vi "HFRR ADV v12.vi"() -> ()   [LabVIEW 2025] (continued)
            n428 = call "IMAGE PATH CREATION PY.vi"("error in (no error)"=w659, "File Name :"=w660) -> ("error out"=w658:errorcluster, "File Path"=w646:path, "File Path String:"=w641:string)  [unwired: 7 in]
            n429 = Match Pattern(string=w654, regular expression=",") -> (before substring=w640:string)  [unwired: 1 in, 3 out]
            n430 = local read "Calibration Tab"() -> (w643:enum32{"Measrument", "Calibrate"})
            n431 = call "Stall Data Flow.vim"("value in"=w658, "milliseconds to wait"=u32 250) -> ("value out"=w642:errorcluster)  [unwired: 1 out]
            n432 = Equal?(x=w640, y="\"rectangle\"") -> (x = y?=w651:bool)
            n433 = case shown="False" w651 {
              tunnel: w650 -> [w705 w760]
              tunnel: w647 -> [_ w751]
              tunnel: cluster{"major":dbl, "minor":dbl, "average":dbl} {"major"=0.0, "minor"=0.0, "average"=0.0} -> [w703 w747]
              tunnel: [w702 w744] -> w645
              tunnel: w640 -> [w704 _]
              tunnel: w647 -> [w701 _]
              frame False {
                n434 = Equal?(x=w704, y="\"line\"") -> (x = y?=w706:bool)
                n435 = case shown="True" w706 {
                  tunnel: w705 -> [_ w721]
                  tunnel: w703 -> [w708 w720]
                  tunnel: [w708 w718] -> w702
                  tunnel: w701 -> [_ w717]
                  frame False {
                  }
                  frame True {
                    w716 = 0.0 ("Major Axis")
                    n436 = Match Pattern(string=w721, regular expression="\"length_px\":") -> (after substring=w719:string)  [unwired: 1 in, 3 out]
                    n437 = property on="Major Axis" class="DigNum (strict)"("Caption.Text"="") -> ()  [unwired: 2 in, 2 out]
                    n438 = property on="Minor Axis" class="DigNum (strict)"("Caption.Text"="") -> ()  [unwired: 2 in, 2 out]
                    n439 = property on="Average" class="DigNum (strict)"("Caption.Text"="Line") -> ()  [unwired: 2 in, 2 out]
                    n440 = Fract/Exp String To Number(string=w719, default (0 dbl)=0.0 ("default (0 DBL)")) -> (number=w715:dbl)  [unwired: 2 in, 1 out]
                    "Pixel Value" <- w715
                    n441 = Multiply(x=w715, y=w717) -> (x*y=w728:dbl)
                    n442 = Multiply(x=w728, y=1000.0) -> (x*y=w711:dbl)
                    n443 = Divide(x=w711, y=1000.0) -> (x/y=w714:dbl)
                    n444 = local write "Measurment (mm)"(w714) -> ()
                    n445 = Bundle By Name(cluster=w720, "average"=w711) -> (w718:cluster{"major":dbl, "minor":dbl, "average":dbl})
                    n446 = Number To Fractional String(number=w711, precision (6)=i16 1) -> (F-format string=w710:string)  [unwired: 2 in]
                    n447 = local write "Minor Axis"(w716) -> ()
                    n448 = local write "Major Axis"(w716) -> ()
                    n449 = Fract/Exp String To Number(string=w710) -> (number=w709:dbl)  [unwired: 3 in, 1 out]
                    n450 = local write "Average"(w709) -> ()
                  }
                }
              }
              frame True {
                w748 = 1000.0 ("y")
                w754 = 0.0 ("default (0 DBL)")
                n451 = Match Pattern(string=w760, regular expression=" \"width_px\":") -> (after substring=w758:string)  [unwired: 1 in, 3 out]
                n452 = Match Pattern(string=w758, regular expression="\"height_px\":") -> (before substring=w756:string, after substring=w755:string)  [unwired: 1 in, 2 out]
                n453 = Fract/Exp String To Number(string=w756, default (0 dbl)=w754) -> (number=w753:dbl)  [unwired: 2 in, 1 out]
                n454 = Fract/Exp String To Number(string=w755, default (0 dbl)=w754) -> (number=w752:dbl)  [unwired: 2 in, 1 out]
                n455 = Multiply(x=w753, y=w751) -> (x*y=w750:dbl)
                n456 = Multiply(x=w752, y=w751) -> (x*y=w749:dbl)
                n457 = Multiply(x=w750, y=w748) -> (x*y=w734:dbl)
                n458 = Multiply(x=w749, y=w748) -> (x*y=w732:dbl)
                n459 = Add(x=w734, y=w732) -> (x+y=w746:dbl)
                n460 = property on="Major Axis" class="DigNum (strict)"("Caption.Text"="Major Axis") -> ()  [unwired: 2 in, 2 out]
                n461 = property on="Minor Axis" class="DigNum (strict)"("Caption.Text"="Minor Axis") -> ()  [unwired: 2 in, 2 out]
                n462 = property on="Average" class="DigNum (strict)"("Caption.Text"="Average") -> ()  [unwired: 2 in, 2 out]
                n463 = Divide(x=w746, y=2.0) -> (x/y=w730:dbl)
                n464 = Bundle By Name(cluster=w747, "major"=w734, "minor"=w732, "average"=w730) -> (w744:cluster{"major":dbl, "minor":dbl, "average":dbl})
                n465 = Number To Fractional String(number=w732, precision (6)=i16 1) -> (F-format string=w739:string)  [unwired: 2 in]
                n466 = Number To Fractional String(number=w730, precision (6)=i16 1) -> (F-format string=w740:string)  [unwired: 2 in]
                n467 = Number To Fractional String(number=w734, precision (6)=i16 1) -> (F-format string=w738:string)  [unwired: 2 in]
                n468 = Fract/Exp String To Number(string=w739) -> (number=w731:dbl)  [unwired: 3 in, 1 out]
                n469 = Fract/Exp String To Number(string=w740) -> (number=w729:dbl)  [unwired: 3 in, 1 out]
                n470 = Fract/Exp String To Number(string=w738) -> (number=w733:dbl)  [unwired: 3 in, 1 out]
                n471 = local write "Major Axis"(w733) -> ()
                n472 = local write "Average"(w729) -> ()
                n473 = local write "Minor Axis"(w731) -> ()
              }
            }
            n474 = case shown="\"Measrument\", Default" w643 {
              tunnel: w646 -> [w673 _]
              tunnel: w645 -> [w672 _]
              tunnel: [w669 w698] -> w644
              tunnel: w642 -> [w671 w698]
              tunnel: w641 -> [w670 _]
              tunnel: w638 -> [w668 _]
              frame "Measrument", Default {
                n475 = stacked-sequence {
                  tunnel: w673 -> [w691 _]
                  tunnel: w672 -> [w689 _]
                  tunnel: w671 -> [w687 _]
                  tunnel: w670 -> [w686 _]
                  tunnel: [w681 _] -> w669
                  tunnel: w668 -> [w674 _]
                  frame #0 {
                    n476 = call "IMAGE ANALYSIS.vi"("Enum"=POST_ANALYSIS_ENUM."SAVE IMAGE", "error in"=w687, "IMAGE FILE PATH"=w686) -> ("error out"=w685:errorcluster)  [unwired: 7 in, 1 out]
                    n477 = call "Stall Data Flow.vim"("value in"=w685, "milliseconds to wait"=u32 1000) -> ("value out"=w676:errorcluster)  [unwired: 1 out]
                    n478 = local read "Test File List :"() -> (w693:string)
                    n479 = call "IMAGE ANALYSIS.vi"("Enum"=POST_ANALYSIS_ENUM."MINIMIZE UI", "error in"=w676) -> ("error out"=w683:errorcluster)  [unwired: 8 in, 1 out]
                    n480 = Bundle By Name(cluster=T21 {"File Name"="", "Test Method"="", "Operator"="", "Fuel Description"="", "Date and time"=""} ("Main Ref"), "Test Method"=w674, "File Name"=w693) -> (w694:T21)
                    n481 = call "Stall Data Flow.vim"("value in"=w683, "milliseconds to wait"=u32 1500) -> ("value out"=w678:errorcluster)  [unwired: 1 out]
                    n482 = call "duf file read.vi"("error in (no error)"=w678, "Main Ref"=w694) -> ("error out"=w692:errorcluster, "Main Ref 2"=w690:T21)  [unwired: 8 in]
                    n483 = call "DETECTION REPORT for manual.vi"("error in (no error)"=w692, "return value 3"=w689, "Image File Path"=w691, "Main Ref"=w690) -> ("error out"=w688:errorcluster)  [unwired: 7 in]
                    n484 = call <vilib>:"Clear Errors.vi"("error in (no error)"=w688) -> ("error out"=w679:errorcluster)  [unwired: 5 in, 1 out]
                    n485 = call "IMAGE ANALYSIS.vi"("Enum"=POST_ANALYSIS_ENUM."MINIMIZE UI", "error in"=w679) -> ("error out"=w681:errorcluster)  [unwired: 8 in, 1 out]
                  }
                  frame #1 {
                    n486 = local write "Main Tab"(T2."HOME" ("Main Tab")) -> ()
                    n487 = local write "Main Dashboard Buttons"(T1."Home" ("Main Dashboard Buttons")) -> ()
                  }
                }
              }
              frame "Calibrate" {
              }
            }
          }
          frame #2 {
            n488 = Not(x=w763) -> (.not. x?=w762:bool)
            n489 = local write "Confirm Measrurement"(w762) -> ()
            n490 = local read "Calibration Tab"() -> (w761:enum32{"Measrument", "Calibrate"})
            n491 = case shown="\"Measrument\", Default" w761 {
              frame "Measrument", Default {
                n492 = local write "Main Tab"(T2."HOME" ("Main Tab")) -> ()
              }
              frame "Calibrate" {
              }
            }
          }
        }
      }
    }
    n493 = local read "Humidity"() -> (w506:bool)
    n494 = local read "Save Change"() -> (w511:bool)
    n495 = local read "Calibrate"() -> (w512:bool)
    n496 = local read "Auto Start Test"() -> (w507:bool)
    n497 = case shown="True" w512 {
      selector: w512 -> [_ w619]
      frame False {
      }
      frame True {
        n498 = Not(x=w619) -> (.not. x?=w618:bool)
        n499 = local write "Calibrate"(w618) -> ()
        n500 = local write "Calibration Tab"(enum32{"Measrument", "Calibrate"}."Calibrate" ("Calibration Tab")) -> ()
      }
    }
    n501 = case shown="True" w511 {
      selector: w511 -> [_ w563]
      frame False {
      }
      frame True {
        n502 = stacked-sequence {
          tunnel: w563 -> [_ _ _ _ w617]
          frame #0 {
            n503 = call "IMAGE ANALYSIS.vi"("Enum"=POST_ANALYSIS_ENUM."HIDE UI") -> ()  [unwired: 9 in, 2 out]
          }
          frame #1 {
            n504 = local read "100x gain"() -> (w565:dbl)
            n505 = local read "10x Gain"() -> (w566:dbl)
            n506 = local read "5x Gain"() -> (w567:dbl)
            n507 = Number To Fractional String(number=w566, width (-)=i16 4, precision (6)=i16 7) -> (F-format string=w588:string)  [unwired: 1 in]
            n508 = Number To Fractional String(number=0.0, width (-)=i16 4, precision (6)=i16 7) -> (F-format string=w583:string)  [unwired: 1 in]
            n509 = Number To Fractional String(number=w565, width (-)=i16 4, precision (6)=i16 7) -> (F-format string=w571:string)  [unwired: 1 in]
            n510 = Number To Fractional String(number=w567, width (-)=i16 10 ("precision (6)"), precision (6)=i16 7) -> (F-format string=w597:string)  [unwired: 1 in]
            n511 = Concatenate Strings("[CH1]" ("string"), w597, " - 5x Gain" ("string"), "\r") -> (w587:string)
            n512 = Concatenate Strings("[CH2]" ("string"), w588, " - 10x Gain" ("string"), "\r") -> (w586:string)
            n513 = Concatenate Strings("[CH3]" ("string"), w583, " - 20x Gain" ("string"), "\r") -> (w577:string)
            n514 = Concatenate Strings("[CH4]" ("string"), w571, " - 100x Gain" ("string"), "\r") -> (w570:string)
            n515 = String To Path(string="C:\\LAB-IQ\\Image Calibrate v01.dcf") -> (path=w600:path)
            n516 = Concatenate Strings(w587, w586, w577, w570) -> (w585:string)
            n517 = call <vilib>:"Write Characters To File.vi"("append to file? (new file:F)"=FALSE, "character string"=w585, "file path (dialog if empty)"=w600) -> ()  [unwired: 2 in, 1 out]
          }
          frame #2 {
            n518 = String To Path(string="C:\\LAB-IQ\\Image Calibrate v01.dcf") -> (path=w603:path)
            n519 = Open/Create/Replace File ("Open File")(file path (use dialog)=w603) -> (refnum out=w604:refnum<file>)  [unwired: 5 in, 2 out]
            n520 = for {
              N: 4 -> [_]
              tunnel: w604 -> [w610]
              i -> [w606]
              n521 = Read from Text File ("Read File")(file (use dialog)=w610) -> (text=w611:string)  [unwired: 3 in, 3 out]
              n522 = String Subset(string=w611, offset (0)=6, length (rest)=10 ("length (rest)")) -> (substring=w607:string)
              n523 = Fract/Exp String To Number(string=w607) -> (number=w605:dbl)  [unwired: 3 in, 1 out]
              n524 = case shown="3" w606 {
                tunnel: w605 -> [w612 w613 _ w614 _]
                frame 0 {
                  n525 = local write "5x Gain"(w612) -> ()
                }
                frame 1 {
                  n526 = local write "10x Gain"(w613) -> ()
                }
                frame 2 {
                }
                frame 3 {
                  n527 = local write "100x gain"(w614) -> ()
                }
                frame 4, Default {
                }
              }
            }
          }
          frame #3 {
            n528 = call "IMAGE ANALYSIS.vi"("Enum"=POST_ANALYSIS_ENUM."SHOW UI") -> ()  [unwired: 9 in, 2 out]
          }
          frame #4 {
            n529 = Not(x=w617) -> (.not. x?=w616:bool)
            n530 = local write "Save Change"(w616) -> ()
          }
        }
      }
    }
    n531 = case shown="False" w507 {
      tunnel: w506 -> [w533 _]
      frame False {
        n532 = case shown="True" w533 {
          frame False {
          }
          frame True {
            n533 = local read "Set Humidity:"() -> (w537:dbl)
            n534 = local read "Set Humidity:"() -> (w540:dbl)
            n535 = local read "Humidity ( %RH )"() -> (w541:dbl)
            n536 = Subtract(x=w537, y=2.0) -> (x-y=w535:dbl)
            n537 = Add(x=w540, y=2.0) -> (x+y=w536:dbl)
            n538 = In Range and Coerce(upper limit=w536, x=w541, lower limit=w535) -> (In Range?=w534:bool)  [unwired: 1 out]
            n539 = case shown="True" w534 {
              frame False {
              }
              frame True {
                n540 = case shown="False" "Manual Humididty Reached" {
                  selector: "Manual Humididty Reached" -> [_ w544]
                  frame False {
                  }
                  frame True {
                    n541 = Not(x=w544) -> (.not. x?=w543:bool)
                    n542 = local write "Manual Humididty Reached"(w543) -> ()
                    n543 = local read "EVENT LOG"() -> (w546:string)
                    n544 = call "Event Log.vi"("Content"="Target Humidity reached", "EVENT LOG"=w546) -> ("EVENT LOG"=w545:string)  [unwired: 8 in, 1 out]
                    n545 = local write "EVENT LOG"(w545) -> ()
                  }
                }
              }
            }
          }
        }
      }
      frame True {
        n546 = local write "Manual Humididty Reached"(TRUE ("Manual Humididty Reached")) -> ()
      }
    }
    n547 = local read "Cap Live Image"() -> (w527:bool)
    n548 = local read "SCAR MEASURMENT"() -> (w530:enum32{"Auto Scar", "Manual Scar"})
    n549 = Wait (ms)(milliseconds to wait=u32 250) -> ()  [unwired: 1 out]
    n550 = Equal?(x=w530, y=enum32{"Auto Scar", "Manual Scar"}."Manual Scar" ("SCAR MEASURMENT")) -> (x = y?=w528:bool)
    n551 = And(x=w528, y=w527) -> (x .and. y?=w526:bool)
    n552 = case shown="True" w526 {
      selector: w526 -> [_ w842]
      frame False {
      }
      frame True {
        n553 = stacked-sequence {
          tunnel: [_ _ _ w857 _] -> _
          tunnel: w842 -> [_ _ _ _ w863]
          frame #0 {
            w843 = 0.0
            n554 = local write "Major Axis"(w843) -> ()
            n555 = local write "Minor Axis"(w843) -> ()
            n556 = local write "Average"(w843) -> ()
          }
          frame #1 {
            n557 = call "CAMERA LIVE FEED FGV.vi"("Enum - Menu"=CAMERA_LIVE_FEED_ENUM."CAMERA MINIMIZE") -> ()  [unwired: 9 in, 2 out]
          }
          frame #2 {
            n558 = local read "FILE 3"() -> (w851:string)
            n559 = call <vilib>:"Trim Whitespace.vi"("string"="C:\\LAB-IQ\\images\\") -> ("trimmed string"=w853:string)  [unwired: 1 in]
            n560 = String To Path(string=w853) -> (path=w852:path)
            n561 = Concatenate Strings(w851, ".png" ("string")) -> (w850:string)
            n562 = Build Path(base path=w852, name or relative path=w850) -> (appended path=w848:path)
            n563 = Path To String(path=w848) -> (string=w847:string)
            n564 = call "CAMERA LIVE FEED FGV.vi"("Enum - Menu"=CAMERA_LIVE_FEED_ENUM."CAMERA SAVE", "Image Path"=w847) -> ("error out"=w845:errorcluster)  [unwired: 8 in, 1 out]
            n565 = case shown="No Error" w845 {
              frame No Error {
                n566 = One Button Dialog(message="Image saved successfully") -> ()  [unwired: 1 in, 1 out]
              }
              frame Error {
              }
            }
          }
          frame #3 {
            n567 = call "LIST FILE NAMES.vi"() -> ("error out"=w859:errorcluster, "filenames"=w856:string[])  [unwired: 10 in]
            n568 = call "IMAGE ANALYSIS.vi"("Enum"=POST_ANALYSIS_ENUM."SHOW UI", "error in"=w859) -> ("error out"=w857:errorcluster)  [unwired: 8 in, 1 out]
            n569 = property on="Test File List :" class="CmbBox"("Strings[]"=w856) -> ()  [unwired: 2 in, 2 out]
          }
          frame #4 {
            (unwired) T22."Report" ("Main Dashboard Buttons")
            n570 = Not(x=w863) -> (.not. x?=w862:bool)
            n571 = local write "Zoom Factore"(0.0 ("Zoom Factore")) -> ()
            n572 = local write "Cap Live Image"(w862) -> ()
            n573 = local write "Main Tab"(T2."Adv Scar Report" ("Main Tab")) -> ()
            n574 = property on="Cap Live Image" class="Bool (strict)"("BoolText.Text"="Capture Image" ("Boolean Text.Text")) -> ()  [unwired: 2 in, 2 out]
            n575 = local write "Main Dashboard Buttons"(T1."Report" ("Main Dashboard Buttons")) -> ()
          }
        }
      }
    }
    n576 = local read "change Gain"() -> (w510:bool)
    n577 = local read "Back Square"() -> (w509:bool)
    n578 = case shown="True" w510 {
      selector: w510 -> [_ w554]
      frame False {
      }
      frame True {
        n579 = stacked-sequence {
          tunnel: w554 -> [_ w562]
          frame #0 {
            n580 = local read "Actual (µm)"() -> (w558:dbl)
            n581 = local read "Pixel Value"() -> (w557:dbl)
            n582 = local read "Magnification :"() -> (w556:string)
            n583 = Divide(x=w558, y=w557) -> (x/y=w555:dbl)
            n584 = case shown="\"10x\"" w556 {
              tunnel: w555 -> [w559 w560]
              frame "10x" {
                n585 = local write "10x Gain"(w559) -> ()
              }
              frame "5x", Default {
                n586 = local write "5x Gain"(w560) -> ()
              }
            }
          }
          frame #1 {
            n587 = Not(x=w562) -> (.not. x?=w561:bool)
            n588 = local write "change Gain"(w561) -> ()
          }
        }
      }
    }
    n589 = case shown="True" w509 {
      selector: w509 -> [_ w552]
      frame False {
      }
      frame True {
        n590 = Not(x=w552) -> (.not. x?=w551:bool)
        n591 = local write "Back Square"(w551) -> ()
        n592 = local write "Calibration Tab"(enum32{"Measrument", "Calibrate"}."Measrument" ("Calibration Tab")) -> ()
      }
    }
    n593 = local read "Rectangle Tool"() -> (w521:bool)
    n594 = local read "Clear ROI Tool"() -> (w520:bool)
    n595 = local read "Open Image"() -> (w525:bool)
    n596 = local read "line tool"() -> (w522:bool)
    n597 = local read "OUT"() -> (w523:bool)
    n598 = local read "In"() -> (w524:bool)
    n599 = case shown="True" w525 {
      selector: w525 -> [_ w830]
      tunnel: [w826 w832] -> _
      tunnel: w515 -> [w826 w831]
      frame False {
      }
      frame True {
        n600 = Not(x=w830) -> (.not. x?=w829:bool)
        n601 = local write "Open Image"(w829) -> ()
        n602 = call "IMAGE ANALYSIS.vi"("Enum"=POST_ANALYSIS_ENUM."HIDE UI", "error in"=w831) -> ("error out"=w839:errorcluster)  [unwired: 8 in, 1 out]
        n603 = call "File Dialog"("start path"=path "C:/LAB-IQ/images", "error in"=w839) -> ("selected path"=w828:path, "error out"=w837:errorcluster)  [unwired: 10 in, 2 out]
        "Image path  2" <- w828
        n604 = call <vilib>:"Clear Errors.vi"("error in (no error)"=w837) -> ("error out"=w836:errorcluster)  [unwired: 5 in, 1 out]
        n605 = call "IMAGE ANALYSIS.vi"("Enum"=POST_ANALYSIS_ENUM."OPEN FILE", "error in"=w836, "File Path"=w828) -> ("error out"=w835:errorcluster)  [unwired: 7 in, 1 out]
        n606 = call <vilib>:"Clear Errors.vi"("error in (no error)"=w835) -> ("error out"=w834:errorcluster)  [unwired: 5 in, 1 out]
        n607 = call "IMAGE ANALYSIS.vi"("Enum"=POST_ANALYSIS_ENUM."SHOW UI", "error in"=w834) -> ("error out"=w832:errorcluster)  [unwired: 8 in, 1 out]
        n608 = local write "Zoom Factore"(100.0 ("Zoom Factore")) -> ()
      }
    }
    n609 = case shown="True" w523 {
      selector: w523 -> [_ w811]
      tunnel: w515 -> [w808 w816]
      tunnel: [w808 w810] -> _
      frame False {
      }
      frame True {
        n610 = Not(x=w811) -> (.not. x?=w809:bool)
        n611 = local read "Zoom Factore"() -> (w814:dbl)
        n612 = local write "OUT"(w809) -> ()
        n613 = call "IMAGE ANALYSIS.vi"("Enum"=POST_ANALYSIS_ENUM."ZOOM OUT", "error in"=w816) -> ("error out"=w810:errorcluster)  [unwired: 8 in, 1 out]
        n614 = Divide(x=w814, y=1.2) -> (x/y=w812:dbl)
        n615 = local write "Zoom Factore"(w812) -> ()
      }
    }
    n616 = case shown="True" w524 {
      selector: w524 -> [_ w820]
      tunnel: w515 -> [w817 w825]
      tunnel: [w817 w818] -> _
      frame False {
      }
      frame True {
        n617 = Not(x=w820) -> (.not. x?=w819:bool)
        n618 = local read "Zoom Factore"() -> (w823:dbl)
        n619 = local write "In"(w819) -> ()
        n620 = call "IMAGE ANALYSIS.vi"("Enum"=POST_ANALYSIS_ENUM."ZOOM IN", "error in"=w825) -> ("error out"=w818:errorcluster)  [unwired: 8 in, 1 out]
        n621 = Multiply(x=w823, y=1.2) -> (x*y=w821:dbl)
        n622 = local write "Zoom Factore"(w821) -> ()
      }
    }
    n623 = case shown="True" w520 {
      selector: w520 -> [_ w792]
      tunnel: w515 -> [w790 w794]
      tunnel: [w790 w793] -> _
      frame False {
      }
      frame True {
        n624 = Not(x=w792) -> (.not. x?=w791:bool)
        n625 = local write "Clear ROI Tool"(w791) -> ()
        n626 = call "IMAGE ANALYSIS.vi"("Enum"=POST_ANALYSIS_ENUM."CLEAR ROI", "error in"=w794) -> ("error out"=w793:errorcluster)  [unwired: 8 in, 1 out]
      }
    }
    n627 = case shown="True" w522 {
      selector: w522 -> [_ w804]
      tunnel: w515 -> [w802 w807]
      tunnel: [w802 w805] -> _
      frame False {
      }
      frame True {
        n628 = Not(x=w804) -> (.not. x?=w803:bool)
        n629 = local write "line tool"(w803) -> ()
        n630 = call "IMAGE ANALYSIS.vi"("Enum"=POST_ANALYSIS_ENUM."DRAW LINE", "error in"=w807) -> ("error out"=w805:errorcluster)  [unwired: 8 in, 1 out]
      }
    }
    n631 = case shown="True" w521 {
      selector: w521 -> [_ w798]
      tunnel: w515 -> [w796 w800]
      tunnel: [w796 w799] -> _
      frame False {
      }
      frame True {
        n632 = Not(x=w798) -> (.not. x?=w797:bool)
        n633 = local write "Rectangle Tool"(w797) -> ()
        n634 = call "IMAGE ANALYSIS.vi"("Enum"=POST_ANALYSIS_ENUM."DRAW REC", "error in"=w800) -> ("error out"=w799:errorcluster)  [unwired: 8 in, 1 out]
      }
    }
    n635 = local read "SCAR MEASURMENT"() -> (w508:enum32{"Auto Scar", "Manual Scar"})
    n636 = local read "Fit to Screen Tool"() -> (w517:bool)
    n637 = local read "Resize Tool"() -> (w516:bool)
    n638 = case shown="\"Manual Scar\", Default" w508 {
      frame "Auto Scar" {
        n639 = property on="Cap Live Image" class="Bool (strict)"("BoolText.Text"="Report" ("Boolean Text.Text")) -> ()  [unwired: 2 in, 2 out]
      }
      frame "Manual Scar", Default {
        n640 = property on="Cap Live Image" class="Bool (strict)"("BoolText.Text"="Save Image" ("Boolean Text.Text")) -> ()  [unwired: 2 in, 2 out]
      }
    }
    n641 = local read "ROI Color Tool"() -> (w518:bool)
    n642 = local read "Pan Tool"() -> (w519:bool)
    n643 = case shown="True" w519 {
      selector: w519 -> [_ w786]
      tunnel: w515 -> [w784 w788]
      tunnel: [w784 w787] -> _
      frame False {
      }
      frame True {
        n644 = Not(x=w786) -> (.not. x?=w785:bool)
        n645 = call "IMAGE ANALYSIS.vi"("Enum"=POST_ANALYSIS_ENUM."PAN", "error in"=w788) -> ("error out"=w787:errorcluster)  [unwired: 8 in, 1 out]
        n646 = local write "Pan Tool"(w785) -> ()
      }
    }
    n647 = case shown="True" w516 {
      selector: w516 -> [_ w770]
      tunnel: w515 -> [w765 w767]
      tunnel: [w765 w766] -> _
      frame False {
      }
      frame True {
        n648 = Not(x=w770) -> (.not. x?=w769:bool)
        n649 = local write "Resize Tool"(w769) -> ()
        n650 = call "IMAGE ANALYSIS.vi"("Enum"=POST_ANALYSIS_ENUM."RESIZE MODE", "error in"=w767) -> ("error out"=w766:errorcluster)  [unwired: 8 in, 1 out]
      }
    }
    n651 = case shown="True" w517 {
      selector: w517 -> [_ w775]
      tunnel: [w771 w776] -> _
      tunnel: w515 -> [w771 w774]
      frame False {
      }
      frame True {
        n652 = Not(x=w775) -> (.not. x?=w773:bool)
        n653 = local write "Zoom Factore"(100.0 ("Zoom Factore")) -> ()
        n654 = local write "Fit to Screen Tool"(w773) -> ()
        n655 = call "IMAGE ANALYSIS.vi"("Enum"=POST_ANALYSIS_ENUM."FIT", "error in"=w774) -> ("error out"=w776:errorcluster)  [unwired: 8 in, 1 out]
      }
    }
    n656 = case shown="True" w518 {
      selector: w518 -> [_ w781]
      tunnel: [w778 w782] -> _
      tunnel: w515 -> [w778 w779]
      frame False {
      }
      frame True {
        n657 = Not(x=w781) -> (.not. x?=w780:bool)
        n658 = local write "ROI Color Tool"(w780) -> ()
        n659 = call "IMAGE ANALYSIS.vi"("Enum"=POST_ANALYSIS_ENUM."SET ROI COLOR", "error in"=w779) -> ("error out"=w782:errorcluster)  [unwired: 8 in, 1 out]
      }
    }
    n660 = local read "Quit"() -> (w532:bool)
  }
  n661 = while {
    stop <- w866 stop-if-true
    n662 = local read "Image Path"() -> (w869:path)
    n663 = local read "Print 3"() -> (w872:bool)
    n664 = Equal?(x=w869, y=path "") -> (x = y?=w868:bool)
    n665 = Not(x=w868) -> (.not. x?=w867:bool)
    n666 = property on="Print 3" class="Bool (strict)"("Visible"=w867) -> ()  [unwired: 2 in, 2 out]
    n667 = case shown="True" w872 {
      frame False {
        n668 = local write "Rd"(TRUE ("Boolean 7")) -> ()
      }
      frame True {
        n669 = flat-sequence {
          tunnel: [w912] -> w880
          tunnel: [w899] -> w878
          tunnel: [w909] -> w874
          tunnel: w880 -> [w921]
          tunnel: [w921] -> w879
          tunnel: w878 -> [w920]
          tunnel: [w920] -> w877
          tunnel: [w918] -> w876
          tunnel: [w917] -> w875
          tunnel: w874 -> [w917]
          tunnel: w879 -> [w923]
          tunnel: w877 -> [w924]
          tunnel: w876 -> [_]
          tunnel: w875 -> [w922]
          frame #0 {
            n670 = case shown="True" "Rd" {
              frame False {
              }
              frame True {
                n671 = while {
                  tunnel: "abcdefABCDEF" ("string 2") -> [w891]
                  shift-right: [w889] -> w883
                  shift-left: "" -> [w888]
                  i -> [w898]
                  stop <- w897 stop-if-true
                  n672 = Random Number (0-1)() -> (number: 0 to 1=w892:dbl)
                  n673 = Multiply(x=w892, y=62.0) -> (x*y=w894:dbl)
                  n674 = Decrement(x="Length 2") -> (x-1=w887:i16)
                  n675 = To Word Integer(number=w894) -> (16bit integer=w895:i16)
                  n676 = String Subset(string=w891, offset (0)=w895, length (rest)=1 ("length (rest)")) -> (substring=w890:string)
                  n677 = Greater Or Equal?(x=w898, y=w887) -> (x >= y?=w897:bool)
                  n678 = Concatenate Strings(w890, w888) -> (w889:string)
                }
                "String 10" <- w883
                n679 = local write "Rd"(FALSE ("Boolean 7")) -> ()
              }
            }
          }
          frame #1 {
            w910 = "_resized.jpg" ("command line")
            (unwired) ".jpg -resize 320x240 " ("string")
            (unwired) "Choose an Image File" ("prompt")
            # "-resize 1798x425"
            n680 = local read "Image Path"() -> (w904:path)
            n681 = Strip Path(path=w904) -> (stripped path=w899:path, name=w900:string)
            n682 = Match Pattern(string=w900, regular expression=".jpg") -> (before substring=→"before substring 2":string, after substring=→"after substring":string)  [unwired: 1 in, 2 out]
            n683 = Match Pattern(string=w900, regular expression="\\") -> (before substring=w906:string)  [unwired: 1 in, 3 out]
            n684 = Match Pattern(string=w906, regular expression=".jpg") -> (before substring=w905:string)  [unwired: 1 in, 3 out]
            n685 = Concatenate Strings("cmd /c convert " ("string"), w905, ".jpg -resize 320x240  " ("command line"), w905, w910) -> (w913:string)
            n686 = call <vilib>:"System Exec.vi"("run minimized? (F)"=TRUE, "wait until completion? (T)"=TRUE, "working directory"=w899, "command line"=w913) -> ("error out"=w912:errorcluster)  [unwired: 4 in, 3 out]
            "error out 2" <- w912
            n687 = Concatenate Strings(w905, w910) -> (w909:string)
          }
          frame #2 {
            n688 = Wait (ms)(milliseconds to wait=u32 2000 ("millisecond timer value")) -> (millisecond timer value=w918:u32)
          }
          frame #3 {
            n689 = case shown="No Error" w923 {
              tunnel: w924 -> [w927 _]
              tunnel: w922 -> [w925 _]
              frame No Error {
                (unwired) ".jpg" ("string")
                n690 = Path To String(path=w927) -> (string=w931:string)
                n691 = Concatenate Strings(w931, "\\" ("string"), w925) -> (w930:string)
                n692 = String To Path(string=w930) -> (path=w929:path)
                n693 = call <vilib>:"Read JPEG File.vi"("path to JPEG file"=w929) -> ("image data"=w933:T14)  [unwired: 8 in, 2 out]
                "image data" <- w933
                n694 = local write "Print 3"(FALSE ("Print 2")) -> ()
                n695 = call <vilib>:"Draw Flattened Pixmap.vi"("image data"=w933) -> ("new picture"=→"new picture":picture)  [unwired: 8 in]
              }
              frame Error {
              }
            }
          }
        }
      }
    }
    n696 = Wait (ms)(milliseconds to wait=u32 20 ("millisecond timer value")) -> ()  [unwired: 1 out]
    n697 = local read "Quit"() -> (w866:bool)
  }
  n698 = property on="Service Password Log" class="Str"("Visible"=w9) -> ()  [unwired: 2 in, 2 out]
  n699 = property on="Password 3" class="Clust (strict)"("Visible"=w9) -> ()  [unwired: 2 in, 2 out]
  n700 = while {
    tunnel: w30 -> [_]
    tunnel: w13 -> [_]
    stop <- w964 stop-if-true
    # "New Adv Logics"
    n701 = local read "Main Tab"() -> (w943:T2)
    n702 = local read "Main Tab"() -> (w962:T2)
    n703 = local read "Sign In"() -> (w961:bool)
    n704 = case shown="\"Adv Scar\"" w943 {
      frame "HOME", Default {
        n705 = local read "LIVE FEED MIN TEMP"() -> (w1091:bool)
        n706 = local write "LIVE FEED MAX TEMP"(TRUE ("LIVE FEED MAX TEMP")) -> ()
        n707 = local read "CAMERA ROI MIN TEMP"() -> (w1089:bool)
        n708 = case shown="True" w1091 {
          selector: w1091 -> [_ w1098]
          frame False {
          }
          frame True {
            n709 = Not(x=w1098) -> (.not. x?=w1097:bool)
            n710 = local write "LIVE FEED MIN TEMP"(w1097) -> ()
            n711 = call "CAMERA LIVE FEED FGV.vi"("Enum - Menu"=CAMERA_LIVE_FEED_ENUM."CAMERA MINIMIZE") -> ()  [unwired: 9 in, 2 out]
          }
        }
        n712 = case shown="True" w1089 {
          selector: w1089 -> [_ w1095]
          frame False {
          }
          frame True {
            n713 = Not(x=w1095) -> (.not. x?=w1094:bool)
            n714 = local write "CAMERA ROI MIN TEMP"(w1094) -> ()
            n715 = call "IMAGE ANALYSIS.vi"("Enum"=POST_ANALYSIS_ENUM."MINIMIZE UI") -> ()  [unwired: 9 in, 2 out]
          }
        }
        n716 = local write "CAMERA ROI MAX TEMP"(TRUE ("CAMERA ROI MAX TEMP")) -> ()
      }
      frame "Test Setup" {
        n717 = local read "LIVE FEED MIN TEMP"() -> (w1101:bool)
        n718 = local read "CAMERA ROI MIN TEMP"() -> (w1099:bool)
        n719 = local write "LIVE FEED MAX TEMP"(TRUE ("LIVE FEED MAX TEMP")) -> ()
        n720 = case shown="True" w1101 {
          selector: w1101 -> [_ w1108]
          frame False {
          }
          frame True {
            n721 = Not(x=w1108) -> (.not. x?=w1107:bool)
            n722 = local write "LIVE FEED MIN TEMP"(w1107) -> ()
            n723 = call "CAMERA LIVE FEED FGV.vi"("Enum - Menu"=CAMERA_LIVE_FEED_ENUM."CAMERA MINIMIZE") -> ()  [unwired: 9 in, 2 out]
          }
        }
        n724 = case shown="True" w1099 {
          selector: w1099 -> [_ w1105]
          frame False {
          }
          frame True {
            n725 = Not(x=w1105) -> (.not. x?=w1104:bool)
            n726 = local write "CAMERA ROI MIN TEMP"(w1104) -> ()
            n727 = call "IMAGE ANALYSIS.vi"("Enum"=POST_ANALYSIS_ENUM."MINIMIZE UI") -> ()  [unwired: 9 in, 2 out]
          }
        }
        n728 = local write "CAMERA ROI MAX TEMP"(TRUE ("CAMERA ROI MAX TEMP")) -> ()
      }
      frame "Acquire" {
        n729 = local read "LIVE FEED MIN TEMP"() -> (w1111:bool)
        n730 = local write "LIVE FEED MAX TEMP"(TRUE ("LIVE FEED MAX TEMP")) -> ()
        n731 = local read "CAMERA ROI MIN TEMP"() -> (w1109:bool)
        n732 = case shown="True" w1111 {
          selector: w1111 -> [_ w1118]
          frame False {
          }
          frame True {
            n733 = Not(x=w1118) -> (.not. x?=w1117:bool)
            n734 = local write "LIVE FEED MIN TEMP"(w1117) -> ()
            n735 = call "CAMERA LIVE FEED FGV.vi"("Enum - Menu"=CAMERA_LIVE_FEED_ENUM."CAMERA MINIMIZE") -> ()  [unwired: 9 in, 2 out]
          }
        }
        n736 = case shown="True" w1109 {
          selector: w1109 -> [_ w1115]
          frame False {
          }
          frame True {
            n737 = Not(x=w1115) -> (.not. x?=w1114:bool)
            n738 = local write "CAMERA ROI MIN TEMP"(w1114) -> ()
            n739 = call "IMAGE ANALYSIS.vi"("Enum"=POST_ANALYSIS_ENUM."MINIMIZE UI") -> ()  [unwired: 9 in, 2 out]
          }
        }
        n740 = local write "CAMERA ROI MAX TEMP"(TRUE ("CAMERA ROI MAX TEMP")) -> ()
      }
      frame "Adv Scar" {
        n741 = local read "CAMERA ROI MIN TEMP"() -> (w1119:bool)
        n742 = case shown="True" "LIVE FEED MAX TEMP" {
          selector: "LIVE FEED MAX TEMP" -> [_ w1140]
          frame False {
          }
          frame True {
            n743 = Not(x=w1140) -> (.not. x?=w1139:bool)
            n744 = local write "LIVE FEED MAX TEMP"(w1139) -> ()
            n745 = call "CAMERA LIVE FEED FGV.vi"("Enum - Menu"=CAMERA_LIVE_FEED_ENUM."CAMERA RESTORE") -> ("error out"=w1130:errorcluster)  [unwired: 9 in, 1 out]
            n746 = Type Cast(type=30, x=0) -> (*(type *) &x=w1134:i32)
            n747 = Add(x=w1134, y=48) -> (x+y=w1135:i32)
            n748 = call "CAMERA LIVE FEED FGV.vi"("Enum - Menu"=CAMERA_LIVE_FEED_ENUM."CAMERA MODE SET", "error in (no error)"=w1130, "CAMERA MODE"=w1135) -> ("error out"=w1127:errorcluster)  [unwired: 7 in, 1 out]
            n749 = call "CAMERA LIVE FEED FGV.vi"("Enum - Menu"=CAMERA_LIVE_FEED_ENUM."CAMERA GRAY", "error in (no error)"=w1127) -> ("error out"=w1126:errorcluster)  [unwired: 8 in, 1 out]
            n750 = call "LIST FILE NAMES.vi"("error in (no error)"=w1126) -> ("error out"=w1136:errorcluster, "filenames"=w1137:string[])  [unwired: 9 in]
            n751 = property on="FILE 3" class="CmbBox"(error in=w1136, "Strings[]"=w1137) -> ()  [unwired: 1 in, 2 out]
          }
        }
        n752 = case shown="True" w1119 {
          selector: w1119 -> [_ w1125]
          frame False {
          }
          frame True {
            n753 = Not(x=w1125) -> (.not. x?=w1124:bool)
            n754 = local write "CAMERA ROI MIN TEMP"(w1124) -> ()
            n755 = call "IMAGE ANALYSIS.vi"("Enum"=POST_ANALYSIS_ENUM."MINIMIZE UI") -> ()  [unwired: 9 in, 2 out]
          }
        }
        n756 = local write "CAMERA ROI MAX TEMP"(TRUE ("CAMERA ROI MAX TEMP")) -> ()
        "LIVE FEED MIN TEMP" <- TRUE ("LIVE FEED MIN TEMP")
      }
      frame "Adv Scar Report" {
        n757 = local read "CAMERA ROI MAX TEMP"() -> (w1141:bool)
        n758 = local read "LIVE FEED MIN TEMP"() -> (w1143:bool)
        n759 = local write "LIVE FEED MAX TEMP"(TRUE ("LIVE FEED MAX TEMP")) -> ()
        n760 = case shown="True" w1143 {
          selector: w1143 -> [_ w1152]
          frame False {
          }
          frame True {
            n761 = Not(x=w1152) -> (.not. x?=w1151:bool)
            n762 = local write "LIVE FEED MIN TEMP"(w1151) -> ()
            n763 = call "CAMERA LIVE FEED FGV.vi"("Enum - Menu"=CAMERA_LIVE_FEED_ENUM."CAMERA MINIMIZE") -> ()  [unwired: 9 in, 2 out]
          }
        }
        n764 = case shown="True" w1141 {
          selector: w1141 -> [_ w1149]
          frame False {
          }
          frame True {
            n765 = Not(x=w1149) -> (.not. x?=w1147:bool)
            n766 = local write "CAMERA ROI MAX TEMP"(w1147) -> ()
            n767 = call "IMAGE ANALYSIS.vi"("Enum"=POST_ANALYSIS_ENUM."SHOW UI") -> ("error out"=w1146:errorcluster)  [unwired: 9 in, 1 out]
            n768 = call "LIST FILE NAMES.vi"("error in (no error)"=w1146) -> ("filenames"=w1145:string[])  [unwired: 9 in, 1 out]
            n769 = property on="Test File List :" class="CmbBox"("Strings[]"=w1145) -> ()  [unwired: 2 in, 2 out]
          }
        }
        n770 = local write "CAMERA ROI MIN TEMP"(TRUE ("CAMERA ROI MIN TEMP")) -> ()
      }
      frame "Compare Files" {
        n771 = local read "LIVE FEED MIN TEMP"() -> (w1155:bool)
        n772 = local write "LIVE FEED MAX TEMP"(TRUE ("LIVE FEED MAX TEMP")) -> ()
        n773 = local read "CAMERA ROI MIN TEMP"() -> (w1153:bool)
        n774 = case shown="True" w1155 {
          selector: w1155 -> [_ w1162]
          frame False {
          }
          frame True {
            n775 = Not(x=w1162) -> (.not. x?=w1161:bool)
            n776 = local write "LIVE FEED MIN TEMP"(w1161) -> ()
            n777 = call "CAMERA LIVE FEED FGV.vi"("Enum - Menu"=CAMERA_LIVE_FEED_ENUM."CAMERA MINIMIZE") -> ()  [unwired: 9 in, 2 out]
          }
        }
        n778 = case shown="True" w1153 {
          selector: w1153 -> [_ w1159]
          frame False {
          }
          frame True {
            n779 = Not(x=w1159) -> (.not. x?=w1158:bool)
            n780 = local write "CAMERA ROI MIN TEMP"(w1158) -> ()
            n781 = call "IMAGE ANALYSIS.vi"("Enum"=POST_ANALYSIS_ENUM."MINIMIZE UI") -> ()  [unwired: 9 in, 2 out]
          }
        }
        n782 = local write "CAMERA ROI MAX TEMP"(TRUE ("CAMERA ROI MAX TEMP")) -> ()
      }
      frame "About" {
        n783 = local read "LIVE FEED MIN TEMP"() -> (w1165:bool)
        n784 = local write "LIVE FEED MAX TEMP"(TRUE ("LIVE FEED MAX TEMP")) -> ()
        n785 = local read "CAMERA ROI MIN TEMP"() -> (w1164:bool)
        n786 = case shown="True" w1165 {
          selector: w1165 -> [_ w1172]
          frame False {
          }
          frame True {
            n787 = Not(x=w1172) -> (.not. x?=w1171:bool)
            n788 = local write "LIVE FEED MIN TEMP"(w1171) -> ()
            n789 = call "CAMERA LIVE FEED FGV.vi"("Enum - Menu"=CAMERA_LIVE_FEED_ENUM."CAMERA MINIMIZE") -> ()  [unwired: 9 in, 2 out]
          }
        }
        n790 = case shown="True" w1164 {
          selector: w1164 -> [_ w1169]
          frame False {
          }
          frame True {
            n791 = Not(x=w1169) -> (.not. x?=w1168:bool)
            n792 = local write "CAMERA ROI MIN TEMP"(w1168) -> ()
            n793 = call "IMAGE ANALYSIS.vi"("Enum"=POST_ANALYSIS_ENUM."MINIMIZE UI") -> ()  [unwired: 9 in, 2 out]
          }
        }
        n794 = local write "CAMERA ROI MAX TEMP"(TRUE ("CAMERA ROI MIN TEMP")) -> ()
      }
      frame "Advance" {
        n795 = local read "LIVE FEED MIN TEMP"() -> (w1175:bool)
        n796 = local write "LIVE FEED MAX TEMP"(TRUE ("LIVE FEED MAX TEMP")) -> ()
        n797 = local read "CAMERA ROI MIN TEMP"() -> (w1173:bool)
        n798 = case shown="True" w1175 {
          selector: w1175 -> [_ w1182]
          frame False {
          }
          frame True {
            n799 = Not(x=w1182) -> (.not. x?=w1181:bool)
            n800 = local write "LIVE FEED MIN TEMP"(w1181) -> ()
            n801 = call "CAMERA LIVE FEED FGV.vi"("Enum - Menu"=CAMERA_LIVE_FEED_ENUM."CAMERA MINIMIZE") -> ()  [unwired: 9 in, 2 out]
          }
        }
        n802 = local write "CAMERA ROI MAX TEMP"(TRUE ("CAMERA ROI MAX TEMP")) -> ()
        n803 = case shown="True" w1173 {
          selector: w1173 -> [_ w1179]
          frame False {
          }
          frame True {
            n804 = Not(x=w1179) -> (.not. x?=w1178:bool)
            n805 = local write "CAMERA ROI MIN TEMP"(w1178) -> ()
            n806 = call "IMAGE ANALYSIS.vi"("Enum"=POST_ANALYSIS_ENUM."MINIMIZE UI") -> ()  [unwired: 9 in, 2 out]
          }
        }
      }
      frame "Mooha" {
        n807 = local read "LIVE FEED MIN TEMP"() -> (w1185:bool)
        n808 = local write "LIVE FEED MAX TEMP"(TRUE ("LIVE FEED MAX TEMP")) -> ()
        n809 = local read "CAMERA ROI MIN TEMP"() -> (w1183:bool)
        n810 = case shown="True" w1185 {
          selector: w1185 -> [_ w1192]
          frame False {
          }
          frame True {
            n811 = Not(x=w1192) -> (.not. x?=w1191:bool)
            n812 = local write "LIVE FEED MIN TEMP"(w1191) -> ()
            n813 = call "CAMERA LIVE FEED FGV.vi"("Enum - Menu"=CAMERA_LIVE_FEED_ENUM."CAMERA MINIMIZE") -> ()  [unwired: 9 in, 2 out]
          }
        }
        n814 = local write "CAMERA ROI MAX TEMP"(TRUE ("CAMERA ROI MAX TEMP")) -> ()
        n815 = case shown="True" w1183 {
          selector: w1183 -> [_ w1189]
          frame False {
          }
          frame True {
            n816 = Not(x=w1189) -> (.not. x?=w1188:bool)
            n817 = local write "CAMERA ROI MIN TEMP"(w1188) -> ()
            n818 = call "IMAGE ANALYSIS.vi"("Enum"=POST_ANALYSIS_ENUM."MINIMIZE UI") -> ()  [unwired: 9 in, 2 out]
          }
        }
      }
    }
    n819 = local read "Auto Start Test"() -> (w934:bool)
    n820 = case shown="True" "sign in temp" {
      frame False {
      }
      frame True {
        w971 = 1 ("y")
        n821 = local read "USERNAME"() -> (w977:string)
        n822 = local read "USER ID"() -> (w974:string)
        n823 = call <vilib>:"Trim Whitespace.vi"("string"=w977) -> ("trimmed string"=w976:string)  [unwired: 1 in]
        n824 = call <vilib>:"Trim Whitespace.vi"("string"=w974) -> ("trimmed string"=w975:string)  [unwired: 1 in]
        n825 = String Length(string=w976) -> (length=w973:i32)
        n826 = String Length(string=w975) -> (length=w972:i32)
        n827 = Greater?(x=w973, y=w971) -> (0:w970:bool)
        n828 = Greater?(x=w972, y=w971) -> (0:w969:bool)
        n829 = And(x=w970, y=w969) -> (x .and. y?=w968:bool)
        n830 = case shown="True" w968 {
          frame False {
            n831 = property on="Sign In" class="Bool (strict)"("DisabledEnum"=T16."Disabled" ("Disabled")) -> ()  [unwired: 2 in, 2 out]
          }
          frame True {
            n832 = property on="Sign In" class="Bool (strict)"("DisabledEnum"=T16."Enabled" ("Disabled")) -> ()  [unwired: 2 in, 2 out]
          }
        }
      }
    }
    n833 = local read "Air Temperature"() -> (w951:bool)
    n834 = local read "Coefficient Of Friction"() -> (w952:bool)
    n835 = case shown="False" w934 {
      frame False {
        n836 = local read "Auto stop temp"() -> (w965:bool)
        n837 = case shown="True" w965 {
          frame False {
          }
          frame True {
            n838 = local write "Auto Start Temp"(FALSE ("Auto Start Temp")) -> ()
          }
        }
      }
      frame True {
        "Auto stop temp" <- TRUE ("Auto stop temp")
      }
    }
    n839 = local read "Humidity"() -> (w950:bool)
    n840 = case shown="\"HOME\"" w962 {
      frame "HOME" {
        n841 = local write "main tab sub"(enum32{"Page 1", "Page 2"}."Page 1" ("main tab sub")) -> ()
      }
      frame Default {
        n842 = local write "main tab sub"(enum32{"Page 1", "Page 2"}."Page 2" ("main tab sub")) -> ()
      }
    }
    n843 = case shown="True" w961 {
      selector: w961 -> [_ w1297]
      frame False {
      }
      frame True {
        n844 = Not(x=w1297) -> (.not. x?=w1296:bool)
        n845 = local write "Sign In"(w1296) -> ()
        n846 = local write "Main Dashboard Buttons"(T1."Test Setup" ("Main Dashboard Buttons")) -> ()
      }
    }
    n847 = case shown="\"Numeric Display\", Default" "Num/Graph" {
      frame "Numeric Display", Default {
        n848 = property on="Single/Multiple" class="RadioBtnsControl (strict)"("Visible"=FALSE) -> ()  [unwired: 2 in, 2 out]
        n849 = property on="Single - Graph" class="Ring (strict)"("Visible"=FALSE) -> ()  [unwired: 2 in, 2 out]
        n850 = local write "Main Tab Display"(T4."Dashboard 1" ("Main Tab Display")) -> ()
      }
      frame "Graph Display" {
        n851 = property on="Single/Multiple" class="RadioBtnsControl (strict)"("Visible"=TRUE) -> ()  [unwired: 2 in, 2 out]
        n852 = case shown="\"Multiple\"" "Single/Multiple" {
          frame "Single ", Default {
            n853 = property on="Single - Graph" class="Ring (strict)"("Visible"=TRUE) -> ()  [unwired: 2 in, 2 out]
            n854 = local write "Main Tab Display"(T4."Dashboard 3" ("Main Tab Display")) -> ()
          }
          frame "Multiple" {
            n855 = property on="Single - Graph" class="Ring (strict)"("Visible"=FALSE) -> ()  [unwired: 2 in, 2 out]
            n856 = local write "Main Tab Display"(T4."Dashboard 2" ("Main Tab Display")) -> ()
          }
        }
      }
    }
    n857 = local read "Stroke"() -> (w949:bool)
    n858 = local read "USERNAME"() -> (w955:string)
    n859 = local read "USER ID"() -> (w954:string)
    n860 = case shown="True" w952 {
      selector: w952 -> [_ w1232]
      frame False {
      }
      frame True {
        n861 = Not(x=w1232) -> (.not. x?=w1231:bool)
        n862 = local write "Coefficient Of Friction"(w1231) -> ()
        n863 = local write "Tab Control 2"(T6."Coefficient Of Friction" ("Tab Control 2")) -> ()
      }
    }
    n864 = case shown="True" w951 {
      selector: w951 -> [_ w1229]
      frame False {
      }
      frame True {
        n865 = Not(x=w1229) -> (.not. x?=w1227:bool)
        n866 = local write "Air Temperature"(w1227) -> ()
        n867 = local write "Tab Control 2"(T6."Air Temperature" ("Tab Control 2")) -> ()
      }
    }
    n868 = local write "Operator ID"(w954) -> ()
    n869 = case shown="True" w949 {
      selector: w949 -> [_ w1223]
      frame False {
      }
      frame True {
        n870 = Not(x=w1223) -> (.not. x?=w1221:bool)
        n871 = local write "Stroke"(w1221) -> ()
        n872 = local write "Tab Control 2"(T6."Stroke" ("Tab Control 2")) -> ()
      }
    }
    n873 = local write "tested by"(w955) -> ()
    n874 = case shown="True" w950 {
      selector: w950 -> [_ w1226]
      frame False {
      }
      frame True {
        n875 = Not(x=w1226) -> (.not. x?=w1224:bool)
        n876 = local write "Humidity"(w1224) -> ()
        n877 = local write "Tab Control 2"(T6."Humidity" ("Tab Control 2")) -> ()
      }
    }
    n878 = case shown="\"Advance\"" "Main Dashboard Buttons" {
      tunnel: [T2."HOME" ("Main Tab") T2."Test Setup" ("Main Tab") T2."Acquire" ("Main Tab") T2."Adv Scar" ("Main Tab") T2."Adv Scar Report" ("Main Tab") T2."Compare Files" ("Main Tab") T2."About" ("Main Tab") T2."Advance" ("Main Tab")] -> w959
      frame "Home", Default {
      }
      frame "Test Setup" {
      }
      frame "Dashboard" {
      }
      frame "Imaging" {
      }
      frame "Report" {
      }
      frame "Analysis" {
      }
      frame "About" {
      }
      frame "Advance" {
      }
    }
    n879 = Wait (ms)(milliseconds to wait=u32 100) -> ()  [unwired: 1 out]
    n880 = local read "Main Tab Display"() -> (w953:T4)
    n881 = local write "Main Tab"(w959) -> ()
    n882 = case shown="\"Dashboard 3\"" w953 {
      frame "Dashboard 1", Default {
        n883 = property on="Reset Graph" class="Bool (strict)"("Visible"=FALSE) -> ()  [unwired: 2 in, 2 out]
      }
      frame "Dashboard 2" {
        n884 = property on="Reset Graph" class="Bool (strict)"("Visible"=TRUE) -> ()  [unwired: 2 in, 2 out]
      }
      frame "Dashboard 3" {
        n885 = property on="Reset Graph" class="Bool (strict)"("Visible"=TRUE) -> ()  [unwired: 2 in, 2 out]
      }
    }
    n886 = local read "SCAR MEASURMENT"() -> (w941:enum32{"Auto Scar", "Manual Scar"})
    n887 = local read "Humidity"() -> (w956:bool)
    n888 = local read "Cap Live Image"() -> (w938:bool)
    n889 = local read "Sample Temperature"() -> (w948:bool)
    n890 = local read "Air Temp vs Humidity"() -> (w946:bool)
    n891 = local read "Frequency"() -> (w947:bool)
    n892 = case shown="False" w956 {
      frame False {
        n893 = local write "Humidity On Command"(TRUE ("Humidity On Command")) -> ()
        n894 = case shown="True" "Humidity Off Command" {
          selector: "Humidity Off Command" -> [_ w1239]
          frame False {
          }
          frame True {
            n895 = stacked-sequence {
              frame #0 {
                n896 = local read "WriteHumidity"() -> (w1241:string[])
                n897 = Insert Into Array(array=w1241, new element="R;1" ("new element/subarray")) -> (w1242:string[])  [unwired: 1 in]
                n898 = local write "WriteHumidity"(w1242) -> ()
              }
              frame #1 {
                n899 = Wait (ms)(milliseconds to wait=u32 2000) -> ()  [unwired: 1 out]
              }
              frame #2 {
                n900 = local read "EVENT LOG"() -> (w1248:string)
                n901 = local read "WriteHumidity"() -> (w1245:string[])
                n902 = call "Event Log.vi"("Content"="Humidity Control Off" ("string"), "EVENT LOG"=w1248) -> ("EVENT LOG"=w1249:string)  [unwired: 8 in, 1 out]
                n903 = local write "EVENT LOG"(w1249) -> ()
                n904 = Insert Into Array(array=w1245, new element="R;1" ("new element/subarray")) -> (w1246:string[])  [unwired: 1 in]
                n905 = local write "WriteHumidity"(w1246) -> ()
              }
            }
            n906 = Not(x=w1239) -> (.not. x?=w1238:bool)
            n907 = local write "Humidity Off Command"(w1238) -> ()
          }
        }
      }
      frame True {
        n908 = local write "Humidity Off Command"(TRUE ("Humidity Off Command")) -> ()
        n909 = case shown="False" "Humidity On Command" {
          selector: "Humidity On Command" -> [_ w1253]
          frame False {
          }
          frame True {
            n910 = stacked-sequence {
              frame #0 {
                n911 = local read "Set Rh"() -> (w1259:dbl)
                n912 = Number To Fractional String(number=w1259, precision (6)=i16 2) -> (F-format string=w1260:string)  [unwired: 2 in]
                n913 = local read "WriteHumidity"() -> (w1257:string[])
                n914 = Concatenate Strings("M;" ("new element/subarray"), w1260) -> (w1258:string)
                n915 = Insert Into Array(array=w1257, new element=w1258) -> (w1256:string[])  [unwired: 1 in]
                n916 = local write "WriteHumidity"(w1256) -> ()
              }
              frame #1 {
                n917 = Wait (ms)(milliseconds to wait=u32 1500) -> ()  [unwired: 1 out]
              }
              frame #2 {
                (unwired) "% RH" ("string")
                (unwired) i16 2 ("precision (6)")
                (unwired) "M;" ("new element/subarray")
                n918 = local read "Set Rh"() -> (w1267:dbl)
                n919 = Number To Fractional String(number=w1267, precision (6)=i16 2) -> (F-format string=w1264:string)  [unwired: 2 in]
                n920 = local read "WriteHumidity"() -> (w1269:string[])
                n921 = Concatenate Strings("M;" ("new element/subarray"), w1264) -> (w1268:string)
                n922 = Concatenate Strings("Humidity Set to : " ("string"), w1264, "% RH" ("string")) -> (w1262:string)
                n923 = Insert Into Array(array=w1269, new element=w1268) -> (w1270:string[])  [unwired: 1 in]
                n924 = disable-structure shown="Enabled" {
                  frame Enabled {
                    n925 = local read "EVENT LOG"() -> (w1273:string)
                    n926 = call "Event Log.vi"("Content"="Humidity Control On", "EVENT LOG"=w1273) -> ("EVENT LOG"=w1274:string)  [unwired: 8 in, 1 out]
                    n927 = local write "EVENT LOG"(w1274) -> ()
                  }
                  frame Disabled {
                  }
                }
                n928 = disable-structure shown="Enabled" {
                  disable-tunnel: w1262 -> [_ _]
                  frame Enabled {
                    n929 = local read "EVENT LOG"() -> (w1276:string)
                    n930 = call "Event Log.vi"("Content"="Humidity Control On", "EVENT LOG"=w1276) -> ("EVENT LOG"=w1277:string)  [unwired: 8 in, 1 out]
                    n931 = local write "EVENT LOG"(w1277) -> ()
                  }
                  frame Disabled {
                  }
                }
                n932 = local write "WriteHumidity"(w1270) -> ()
              }
            }
            n933 = Not(x=w1253) -> (.not. x?=w1252:bool)
            n934 = local write "Humidity On Command"(w1252) -> ()
          }
        }
      }
    }
    n935 = Equal?(x=w941, y=enum32{"Auto Scar", "Manual Scar"}."Auto Scar" ("SCAR MEASURMENT")) -> (x = y?=w937:bool)
    n936 = local read "TEST STANDARD"() -> (w944:T3)
    n937 = And(x=w938, y=w937) -> (x .and. y?=w939:bool)
    n938 = case shown="True" w939 {
      selector: w939 -> [_ w1038]
      tunnel: errorcluster {"status"=FALSE, "code"=0, "source"=""} ("error in (no error) 3") -> [_ w1039]
      frame False {
      }
      frame True {
        n939 = stacked-sequence {
          tunnel: w1039 -> [_ _ _ _ _ _ _ w1087]
          tunnel: w1038 -> [_ _ _ _ _ w1068 _ _]
          frame #0 {
            n940 = call "CAMERA LIVE FEED FGV.vi"("Enum - Menu"=CAMERA_LIVE_FEED_ENUM."CAMERA MINIMIZE") -> ()  [unwired: 9 in, 2 out]
          }
          frame #1 {
            n941 = property on="Auto Scar Check  2" class="Clust (strict)"("Visible"=TRUE) -> ()  [unwired: 2 in, 2 out]
          }
          frame #2 {
            n942 = String To Path(string="C:\\LAB-IQ\\Image Calibrate v01.dcf") -> (path=w1044:path)
            n943 = Open/Create/Replace File ("Open File")(file path (use dialog)=w1044) -> (refnum out=w1045:refnum<file>)  [unwired: 5 in, 2 out]
            n944 = for {
              N: 4 -> [_]
              tunnel: w1045 -> [w1051]
              i -> [w1047]
              n945 = Read from Text File ("Read File")(file (use dialog)=w1051) -> (text=w1052:string)  [unwired: 3 in, 3 out]
              n946 = String Subset(string=w1052, offset (0)=6, length (rest)=10 ("length (rest)")) -> (substring=w1048:string)
              n947 = Fract/Exp String To Number(string=w1048) -> (number=w1046:dbl)  [unwired: 3 in, 1 out]
              n948 = case shown="0" w1047 {
                tunnel: w1046 -> [w1053 w1054 _ w1055 _]
                frame 0 {
                  "5x Gain" <- w1053
                }
                frame 1 {
                  "10x Gain" <- w1054
                }
                frame 2 {
                }
                frame 3 {
                  "100x gain" <- w1055
                }
                frame 4, Default {
                }
              }
            }
          }
          frame #3 {
            n949 = local read "FILE 3"() -> (w1061:string)
            n950 = call <vilib>:"Trim Whitespace.vi"("string"="C:\\LAB-IQ\\images\\") -> ("trimmed string"=w1063:string)  [unwired: 1 in]
            n951 = String To Path(string=w1063) -> (path=w1062:path)
            n952 = Concatenate Strings(w1061, ".png" ("string")) -> (w1060:string)
            n953 = Build Path(base path=w1062, name or relative path=w1060) -> (appended path=w1058:path)
            "Image path" <- w1058
            n954 = Path To String(path=w1058) -> (string=w1057:string)
            n955 = call "CAMERA LIVE FEED FGV.vi"("Enum - Menu"=CAMERA_LIVE_FEED_ENUM."CAMERA SAVE", "Image Path"=w1057) -> ()  [unwired: 8 in, 2 out]
          }
          frame #4 {
            n956 = One Button Dialog(message="Image saved successfully") -> ()  [unwired: 1 in, 1 out]
          }
          frame #5 {
            n957 = local read "TEST STANDARD"() -> (w1067:T3)
            n958 = local read "Magnification len live scar"() -> (w1079:string)
            n959 = Not(x=w1068) -> (.not. x?=w1069:bool)
            n960 = local write "Cap Live Image"(w1069) -> ()
            n961 = case shown="\"ISO 12156\"" w1067 {
              tunnel: ["ASTM D6079" "ISO 12156"] -> w1066
              frame "ASTM D6079", Default {
              }
              frame "ISO 12156" {
              }
            }
            n962 = case shown="\"5x\", Default" w1079 {
              tunnel: [w1082 w1083] -> w1078
              frame "5x", Default {
                n963 = local read "5x Gain"() -> (w1082:dbl)
              }
              frame "10x" {
                # "5x"
                n964 = local read "10x Gain"() -> (w1083:dbl)
              }
            }
            n965 = local read "Image path"() -> (w1077:path)
            n966 = local read "FILE 3"() -> (w1070:string)
            n967 = call "EDGE DETCTION.vi"("GAIN VALUE"=w1078, "Image Path"=w1077) -> ("error out"=w1076:errorcluster, "return value"=w1075:cluster{string, string, dbl, dbl, dbl})  [unwired: 8 in]
            n968 = Bundle By Name(cluster=T21 {"File Name"="", "Test Method"="", "Operator"="", "Fuel Description"="", "Date and time"=""} ("Main Ref"), "File Name"=w1070, "Test Method"=w1066) -> (w1071:T21)
            n969 = call "duf file read.vi"("error in (no error)"=w1076, "Main Ref"=w1071) -> ("error out"=w1074:errorcluster, "Main Ref 2"=w1072:T21)  [unwired: 8 in]
            n970 = call "EDGE DETECTION REPORT.vi"("error in (no error)"=w1074, "return value 2"=w1075, "Main Ref"=w1072) -> ()  [unwired: 8 in, 1 out]
          }
          frame #6 {
            n971 = property on="Auto Scar Check  2" class="Clust (strict)"("Visible"=FALSE) -> ()  [unwired: 2 in, 2 out]
          }
          frame #7 {
            n972 = call "CAMERA LIVE FEED FGV.vi"("Enum - Menu"=CAMERA_LIVE_FEED_ENUM."CAMERA MINIMIZE", "error in (no error)"=w1087) -> ()  [unwired: 8 in, 2 out]
            n973 = local write "Main Dashboard Buttons"(T1."Home" ("Main Dashboard Buttons")) -> ()
            n974 = local write "Main Tab"(T2."HOME" ("Main Tab")) -> ()
          }
        }
      }
    }
    n975 = local read "Heater Button"() -> (w945:bool)
    n976 = case shown="True" w947 {
      selector: w947 -> [_ w1217]
      frame False {
      }
      frame True {
        n977 = Not(x=w1217) -> (.not. x?=w1215:bool)
        n978 = local write "Frequency"(w1215) -> ()
        n979 = local write "Tab Control 2"(T6."Frequency" ("Tab Control 2")) -> ()
      }
    }
    n980 = case shown="True" w946 {
      selector: w946 -> [_ w1214]
      frame False {
      }
      frame True {
        n981 = Not(x=w1214) -> (.not. x?=w1212:bool)
        n982 = local write "Air Temp vs Humidity"(w1212) -> ()
        n983 = local write "Tab Control 2"(T6."Air Temp vs Rh" ("Tab Control 2")) -> ()
      }
    }
    n984 = case shown="True" w948 {
      selector: w948 -> [_ w1220]
      frame False {
      }
      frame True {
        n985 = Not(x=w1220) -> (.not. x?=w1218:bool)
        n986 = local write "Sample Temperature"(w1218) -> ()
        n987 = local write "Tab Control 2"(T6."Sample Temperature" ("Tab Control 2")) -> ()
      }
    }
    n988 = case shown="\"Custom\"" w944 {
      frame "ASTM D6079", Default {
        w1193 = "ASTM D6079 TEST CONDITIONS" ("Standard 2")
        n989 = local write "Standard 2"(w1193) -> ()
        n990 = local write "Standard"(w1193) -> ()
      }
      frame "ISO 12156" {
        w1194 = "ISO 12156 TEST CONDITIONS" ("Standard 2")
        n991 = local write "Standard 2"(w1194) -> ()
        n992 = local write "Standard"(w1194) -> ()
      }
      frame "CEC F-096-A-06" {
        w1195 = "CEC F-096-A-06 TEST CONDITIONS" ("Standard 2")
        n993 = local write "Standard 2"(w1195) -> ()
        n994 = local write "Standard"(w1195) -> ()
      }
      frame "Custom" {
        w1196 = "CUSTOM TEST CONDITIONS" ("Standard 2")
        n995 = local write "Standard 2"(w1196) -> ()
        n996 = local write "Standard"(w1196) -> ()
      }
    }
    n997 = case shown="True" w945 {
      frame False {
        n998 = local write "Temperature On Command"(TRUE ("Temperature On Command")) -> ()
        n999 = case shown="True" "Temperature Off Command" {
          selector: "Temperature Off Command" -> [_ w1200]
          frame False {
          }
          frame True {
            n1000 = Not(x=w1200) -> (.not. x?=w1199:bool)
            n1001 = local read "EVENT LOG"() -> (w1203:string)
            n1002 = local write "Temperature Off Command"(w1199) -> ()
            n1003 = call "Event Log.vi"("Content"="Heater Off", "EVENT LOG"=w1203) -> ("EVENT LOG"=w1202:string)  [unwired: 8 in, 1 out]
            n1004 = local write "EVENT LOG"(w1202) -> ()
          }
        }
      }
      frame True {
        n1005 = local write "Temperature Off Command"(TRUE ("Temperature Off Command")) -> ()
        n1006 = case shown="True" "Temperature On Command" {
          selector: "Temperature On Command" -> [_ w1207]
          frame False {
          }
          frame True {
            n1007 = Not(x=w1207) -> (.not. x?=w1206:bool)
